vi "Example - Authenticate using multiple methods.vi"() -> ()   [LabVIEW 2020, in "wamplv.lvlib"]
uses:
  wamplv.lvlib
  WAMP Client/WAMP Client.lvclass
  WAMP Client/Private/Authentication/Add ticket authenticator.vi
  WAMP Client/Private/Authentication/Add WAMP-CRA authenticator.vi
panel:
  in  "Ticket secret (e.g. password)":string="secret-ticket"
  in  "WAMP-CRA secret (e.g. password)":string="secret2"
  in  "Authorisation ID (e.g.username)":string="username"
  in  "Arguments":string
  in  "Topic URI":string="test.topic"
  in  "Realm":string="private_realm"
  in  "Router URL":string="ws://192.168.1.10:55555/"
  # "Example: authentcate  with WAMP-CRA or ticket, and publish"
  # "WAMP spec allows for multiple authentication methods,\nbut only a single authorisation ID"
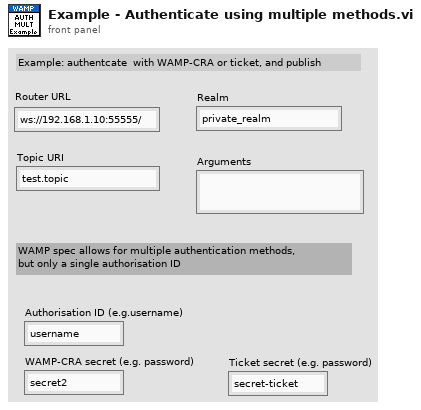
[diagram p1: front panel]
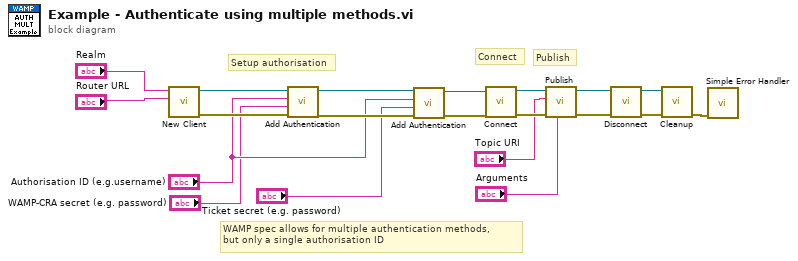
[diagram p0: block diagram]
diagram:
  # "WAMP spec allows for multiple authentication methods,\nbut only a single authorisation ID"
  # "Setup authorisation"
  # "Publish"
  # "Connect"
  n1 = call "New Client.vi"("Address"="Router URL", "Realm"="Realm") -> ("error out"=w8:errorcluster, "WAMP client out"=w9:refnum<class "WAMP Client.lvclass">)  [unwired: 8 in]
  n2 = call-poly "Add Authentication.vi"("error in (no error)"=w8, "Secret"="WAMP-CRA secret (e.g. password)", "Authentication ID"="Authorisation ID (e.g.username)", "WAMP Client in"=w9) -> ("error out"=w6:errorcluster, "WAMP Client out"=w5:refnum<class "WAMP Client.lvclass">)  [unwired: 6 in]
  n3 = call-poly "Add Authentication.vi"("error in (no error)"=w6, "Secret"="Ticket secret (e.g. password)", "Authentication ID"="Authorisation ID (e.g.username)", "WAMP Client in"=w5) -> ("error out"=w7:errorcluster, "WAMP Client out"=w4:refnum<class "WAMP Client.lvclass">)  [unwired: 6 in]
  n4 = call "Connect.vi"("error in"=w7, "WAMP Client in"=w4) -> ("error out"=w13:errorcluster, "WAMP Client out"=w15:refnum<class "WAMP Client.lvclass">)  [unwired: 8 in]
  n5 = call "Publish.vi"("Arguments"="Arguments", "Error in"=w13, "Topic"="Topic URI", "WAMP Client in"=w15) -> ("Error out"=w12:errorcluster, "WAMP Client out"=w14:refnum<class "WAMP Client.lvclass">)  [unwired: 5 in, 1 out]
  n6 = call-dynamic "Disconnect.vi"("error in"=w12, "WAMP Client in"=w14) -> ("error out"=w16:errorcluster, "WAMP Client out"=w18:refnum<class "WAMP Client.lvclass">)  [unwired: 8 in]
  n7 = call-dynamic "Cleanup.vi"("error in"=w16, "WAMP Client in"=w18) -> ("error out"=w17:errorcluster)  [unwired: 8 in, 1 out]
  n8 = call <vilib>:"Simple Error Handler.vi"("error in (no error)"=w17) -> ()  [unwired: 4 in, 5 out]
